vi "실습 1-2 마스트슬레이브.vi"() -> ()   [LabVIEW 2014]
uses:
  <vilib>/Analysis/NI_AALBase.lvlib
panel:
  out "웨이브폼 그래프":dbl[](graph)
  in  "정지":bool
  in  "Send 메시지":bool
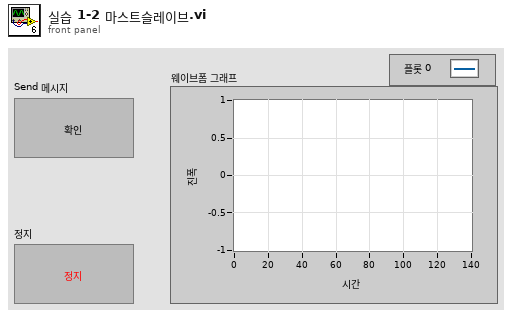
[diagram p1: front panel]
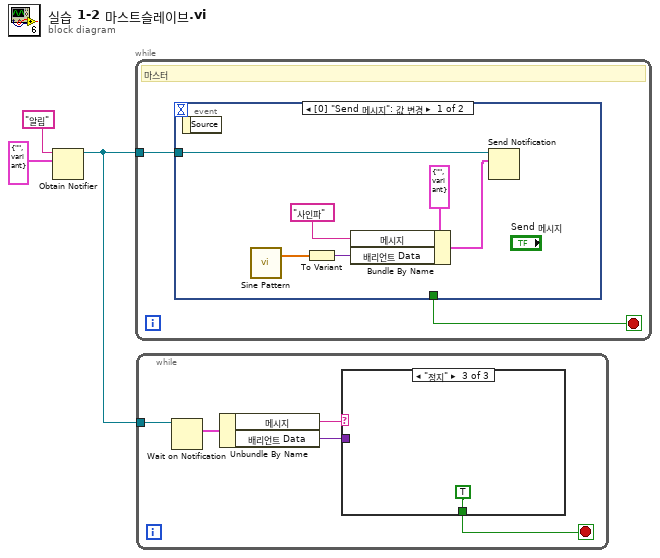
[diagram p0: block diagram]
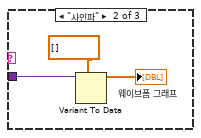
[diagram p3: hidden frame]
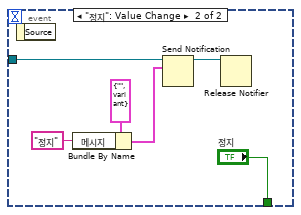
[diagram p4: hidden frame]
diagram:
  n1 = Obtain Notifier(name (unnamed)="알림" ("이름(이름없음)"), notification data type=cluster{"메시지":string, "배리언트 Data":variant} {"메시지"="", "배리언트 Data"=variant} ("알림")) -> (notifier out=w1:refnum<notifier>)  [unwired: 2 in, 2 out]
  n2 = while {
    tunnel: w1 -> [w5]
    stop <- w4 stop-if-true
    # "마스터"
    n3 = event shown="[0] \"Send 메시지\": 값 변경" {
      selector: _ -> [_ _]
      dyn-events: _ -> [_ _]
      timeout: _ -> [_ _]
      tunnel: w5 -> [w7 w16]
      tunnel: [_ "정지"] -> w4
      event "Send 메시지": Value Change {
        n4 = event-data() -> ()  [unwired: 1 in, 1 out]
        n5 = call <vilib>:"Sine Pattern.vi"() -> ("Sinusoidal Pattern"=w8:dbl[])  [unwired: 4 in, 1 out]
        n6 = To Variant(anything=w8) -> (Variant=w9:variant)
        n7 = Bundle By Name(cluster=cluster{"메시지":string, "배리언트 Data":variant} {"메시지"="", "배리언트 Data"=variant} ("알림"), "메시지"="사인파", "배리언트 Data"=w9) -> (w11:cluster{"메시지":string, "배리언트 Data":variant})
        n8 = Send Notification(notification=w11, notifier=w7) -> ()  [unwired: 1 in, 2 out]
      }
      event "정지": Value Change {
        n9 = event-data() -> ()  [unwired: 1 in, 1 out]
        n10 = Bundle By Name(cluster=cluster{"메시지":string, "배리언트 Data":variant} {"메시지"="", "배리언트 Data"=variant} ("알림"), "메시지"="정지") -> (w13:cluster{"메시지":string, "배리언트 Data":variant})
        n11 = Send Notification(notification=w13, notifier=w16) -> (notifier out=w15:refnum<notifier>)  [unwired: 1 in, 1 out]
        n12 = Release Notifier(notifier=w15) -> ()  [unwired: 2 in, 3 out]
      }
    }
  }
  n13 = while {
    tunnel: w1 -> [w22]
    stop <- w19 stop-if-true
    n14 = Wait on Notification(notifier=w22) -> (notification=w21:cluster{"메시지":string, "배리언트 Data":variant})  [unwired: 3 in, 3 out]
    n15 = Unbundle By Name(w21) -> ("메시지"=w20:string, "배리언트 Data"=w18:variant)
    n16 = case shown="\"정지\"" w20 {
      tunnel: [_ _ TRUE] -> w19
      tunnel: w18 -> [_ w24 _]
      frame Default {
      }
      frame "사인파" {
        n17 = Variant To Data(type=dbl[] [] ("Sinusoidal Pattern"), Variant=w24) -> (data=→"웨이브폼 그래프":dbl[])  [unwired: 1 in, 1 out]
      }
      frame "정지" {
      }
    }
  }
